vi "available tag dialog.vi"(7 "channel action event":refnum<user-event>, 8 "error in":errorcluster, 10 "channel to map to":refnum<class "TBM channel.lvclass">, 11 "filtered tags":refnum<class "tag descriptor.lvclass">[](array[class])) -> (0 "error out":errorcluster)   [LabVIEW 2013, in "Table Manager.lvlib"]
uses:
  Table Manager.lvlib
  <vilib>/NI/Tag Bus/tag/tag descriptor.lvclass
  <vilib>/NI/DCAF/Tag Editor Core/control module/editor node/channel action event.ctl
  <vilib>/NI/DCAF/Tag Editor Core/control module/editor node/dialog output action.ctl
  <vilib>/NI/Tag Bus Module Framework/channel/TBM channel.lvclass
  <vilib>/event_ctls.llb/usereventprio.ctl
  <vilib>/NI/Tag Bus/tag/tag descriptor.lvclass/tag descriptor.ctl
  <vilib>/NI/DCAF/Tag Editor Core/control module/editor node/control module editor.lvclass
panel:
  in  "Filter":string
  in  "Available Tags":i32(listbox)
  in  "disconnect":bool
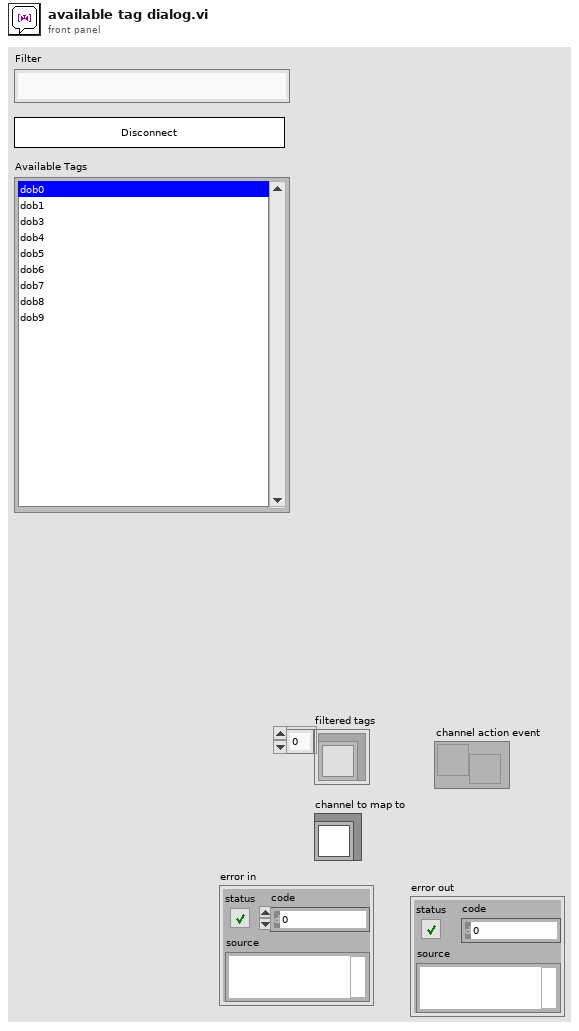
[diagram p1: front panel]
types:
  T1 = typedef "usereventprio.ctl" = enum32{"high priority", "normal priority"}
  T2 = typedef "control module editor.lvclass/dialog output action.ctl" = enum16{"Tag Created", "Tag Selected", "Set Default", "disconnect"}
  T3 = typedef "control module editor.lvclass/channel action event.ctl" = cluster{"action":T2, "channel":refnum<class "TBM channel.lvclass">, "selected tag":refnum<class "tag descriptor.lvclass">}
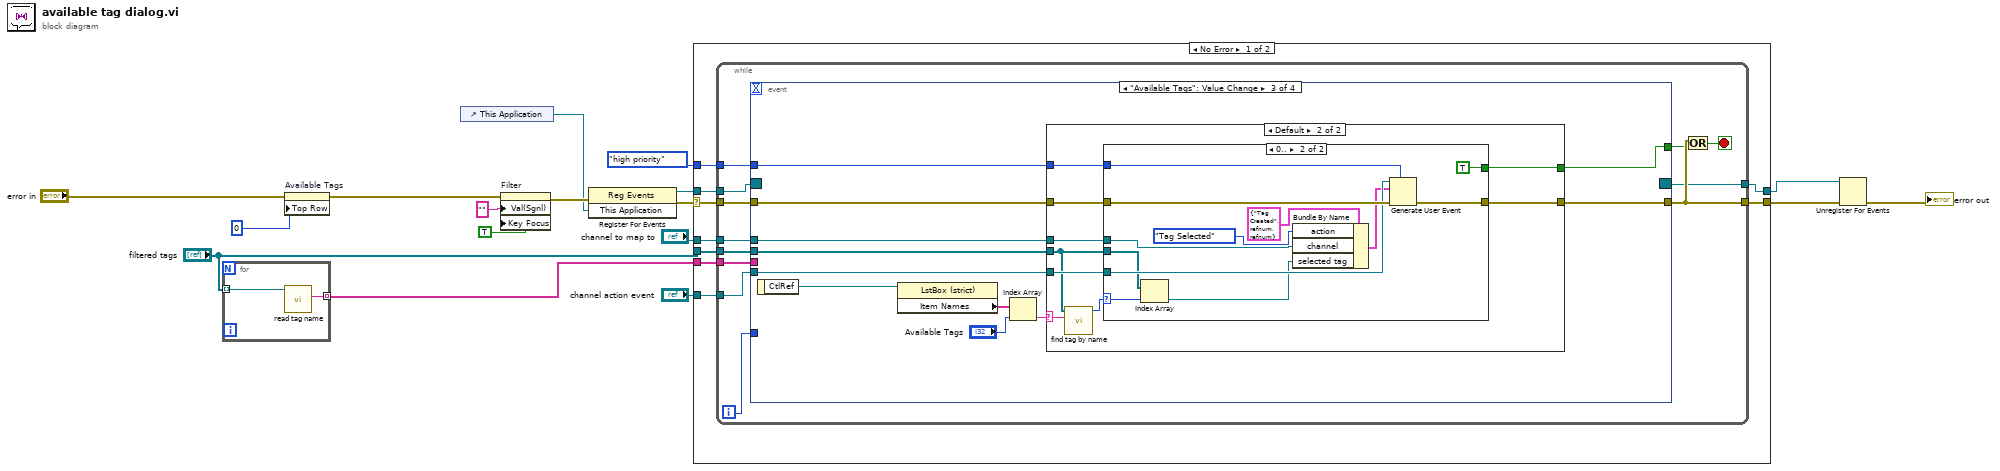
[diagram p0: block diagram]
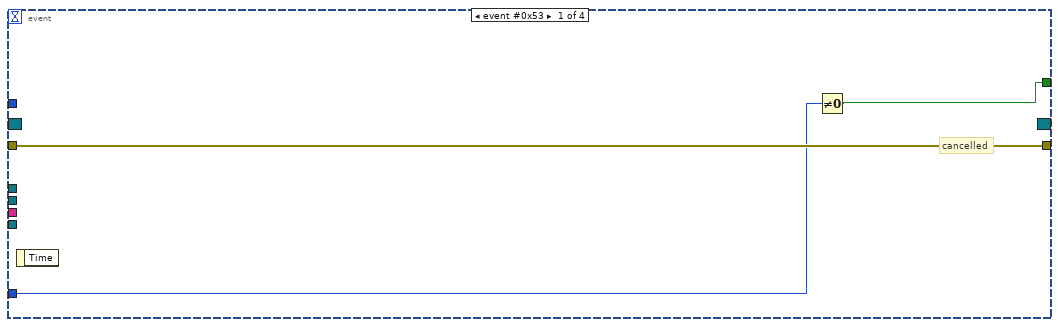
[diagram p2: hidden frame]
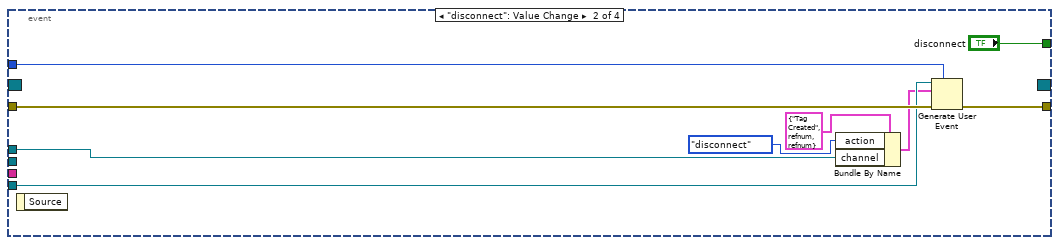
[diagram p3: hidden frame]
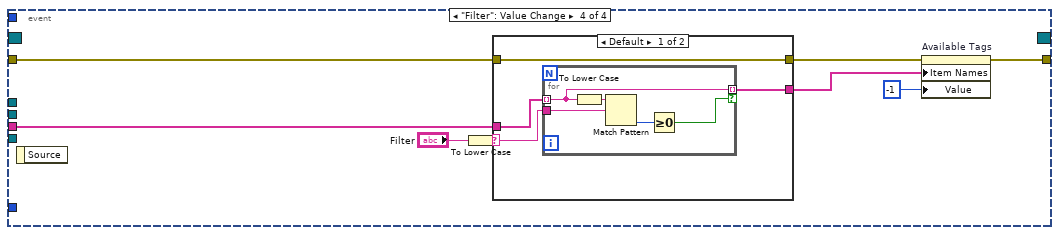
[diagram p6: hidden frame]
diagram:
  n1 = for {
    tunnel: "filtered tags" -> [w19] mode=indexing
    tunnel: [w18] -> w12 mode=indexing
    n2 = call <vilib>:"read tag name.vi"("system tag in"=w19) -> ("name"=w18:string)  [unwired: 8 in, 2 out]
  }
  n3 = property on="Available Tags" class="LstBox (strict)"(error in="error in", "Top Row"=0) -> (error out=w1:errorcluster)  [unwired: 1 in, 1 out]
  n4 = control-ref of="This Application"() -> (w4:refnum<vi>)
  n5 = property on="Filter" class="Str"(error in=w1, "Val(Sgnl)"="" ("Value (Signaling)"), "Key Focus"=TRUE) -> (error out=w11:errorcluster)  [unwired: 1 in, 1 out]
  n6 = register-events(error in=w11, w4) -> (reference out=w7:refnum<event-registration>, error out=w8:errorcluster)  [unwired: 1 in]
  n7 = case shown="No Error" w8 {
    selector: w8 -> [w26 w107]
    tunnel: [w28 w107] -> w17
    tunnel: "channel action event" -> [w27 _]
    tunnel: "channel to map to" -> [w25 _]
    tunnel: usereventprio."high priority" ("priority (normal)") -> [w24 _]
    tunnel: "filtered tags" -> [w23 _]
    tunnel: w12 -> [w22 _]
    tunnel: w7 -> [w21 w106]
    tunnel: [w20 w106] -> w5
    frame No Error {
      n8 = while {
        tunnel: w26 -> [w40]
        tunnel: [w38] -> w28
        tunnel: w27 -> [w36]
        tunnel: w25 -> [w35]
        tunnel: w24 -> [w34]
        tunnel: w23 -> [w33]
        tunnel: w22 -> [w32]
        tunnel: w21 -> [w30]
        tunnel: [w29] -> w20
        i -> [w31]
        stop <- w39 stop-if-true
        n9 = event shown="[2] \"Available Tags\": Value Change" {
          selector: w30 -> [_ _ _ _]
          dyn-events: [_ _ _ _] -> w29
          timeout: _ -> [_ _ _ _]
          tunnel: w40 -> [w43 w52 w63 w94]
          tunnel: [w43 w51 w62 w91] -> w38
          tunnel: [w42 "disconnect" w54 _] -> w37
          tunnel: w36 -> [_ w50 w61 _]
          tunnel: w35 -> [_ w46 w60 _]
          tunnel: w34 -> [_ w45 w59 _]
          tunnel: w33 -> [_ _ w55 _]
          tunnel: w32 -> [_ _ _ w88]
          tunnel: w31 -> [w41 _ _ _]
          event event #0x53 {
            # "cancelled"
            n10 = event-data() -> ()  [unwired: 1 in, 1 out]
            n11 = Not Equal To 0?(x=w41) -> (x != 0?=w42:bool)
          }
          event "disconnect": Value Change {
            n12 = event-data() -> ()  [unwired: 1 in, 1 out]
            n13 = Bundle By Name(cluster=T3 {"action"=enum."Tag Created", "channel"=refnum, "selected tag"=refnum} ("event data"), "action"=dialog_output_action."disconnect", "channel"=w46) -> (w48:T3)
            n14 = Generate User Event(priority (normal)=w45, user event=w50, event data cluster=w48, error in=w52) -> (error out=w51:errorcluster)  [unwired: 1 out]
          }
          event "Available Tags": Value Change {
            n15 = event-data() -> ("CtlRef"=w58:refnum<vi>)  [unwired: 1 in]
            n16 = property class="LstBox (strict)"(reference=w58) -> ("Item Names"=w57:string[])  [unwired: 1 in, 2 out]
            n17 = Index Array(array=w57, index="Available Tags") -> (element=w56:string)
            n18 = case shown="Default" w56 {
              selector: w56 -> [_ w68]
              tunnel: w63 -> [w64 w73]
              tunnel: [w64 w72] -> w62
              tunnel: w61 -> [_ w71]
              tunnel: w60 -> [_ w70]
              tunnel: w59 -> [_ w69]
              tunnel: w55 -> [_ w66]
              tunnel: [_ w65] -> w54
              frame "" {
              }
              frame Default {
                n19 = call <vilib>:"find tag by name.vi"("name"=w68, "tags in"=w66) -> ("index"=w67:i32)  [unwired: 9 in]
                n20 = case shown="0.." w67 {
                  selector: w67 -> [_ w78]
                  tunnel: w73 -> [w74 w86]
                  tunnel: [w74 w85] -> w72
                  tunnel: w71 -> [_ w84]
                  tunnel: w70 -> [_ w80]
                  tunnel: w69 -> [_ w79]
                  tunnel: w66 -> [_ w77]
                  tunnel: [_ TRUE] -> w65
                  frame ..-1 {
                  }
                  frame 0.. {
                    n21 = Index Array(array=w77, index=w78) -> (element=w76:refnum<class "tag descriptor.lvclass">)
                    n22 = Bundle By Name(cluster=T3 {"action"=enum."Tag Created", "channel"=refnum, "selected tag"=refnum} ("event data"), "action"=dialog_output_action."Tag Selected", "channel"=w80, "selected tag"=w76) -> (w82:T3)
                    n23 = Generate User Event(priority (normal)=w79, user event=w84, event data cluster=w82, error in=w86) -> (error out=w85:errorcluster)  [unwired: 1 out]
                  }
                }
              }
            }
          }
          event "Filter": Value Change {
            n24 = event-data() -> ()  [unwired: 1 in, 1 out]
            n25 = To Lower Case(string="Filter") -> (all lower case string=w87:string)
            n26 = case shown="Default" w87 {
              selector: w87 -> [w97 _]
              tunnel: w94 -> [w98 w105]
              tunnel: [w98 w105] -> w90
              tunnel: [w95 w104] -> w89
              tunnel: w88 -> [w96 w104]
              frame Default {
                n27 = for {
                  tunnel: w97 -> [w103]
                  tunnel: w96 -> [w102] mode=indexing
                  tunnel: [w102] -> w95 mode=indexing if=w100
                  n28 = To Lower Case(string=w102) -> (all lower case string=w99:string)
                  n29 = Match Pattern(string=w99, regular expression=w103) -> (offset past match=w101:i32)  [unwired: 1 in, 3 out]
                  n30 = Greater Or Equal To 0?(x=w101) -> (x >= 0?=w100:bool)
                }
              }
              frame "" {
              }
            }
            n31 = property on="Available Tags" class="LstBox (strict)"(error in=w90, "Item Names"=w89, "Value"=-1 ("Available Tags")) -> (error out=w91:errorcluster)  [unwired: 1 in, 1 out]
          }
        }
        n32 = Or(x=w38, y=w37) -> (x .or. y?=w39:bool)
      }
    }
    frame Error {
    }
  }
  n33 = Unregister For Events(event registration refnum=w5, error in=w17) -> (error out=→"error out":errorcluster)
